vi "NT Table Connected AE.vi"(7 "Update":bool, 11 "NT Table Connected in":bool) -> (3 "NT Table Connected out":bool)   [LabVIEW 2025]
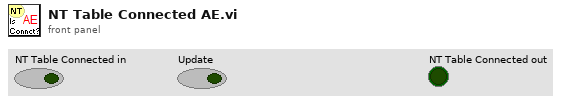
[diagram p1: front panel]
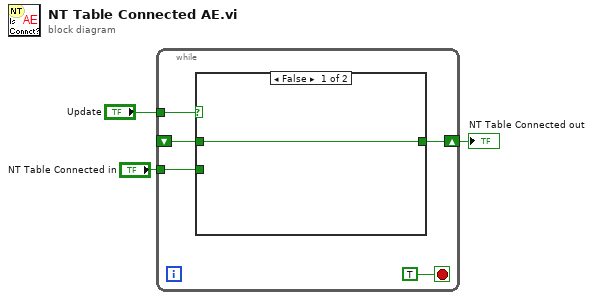
[diagram p0: block diagram]
diagram:
  n1 = while {
    shift-right: [w6] -> w1
    shift-left: _ -> [w4]
    tunnel: "Update" -> [w7]
    tunnel: "NT Table Connected in" -> [w5]
    stop <- TRUE stop-if-true
    n2 = case shown="False" w7 {
      tunnel: [w9 w10] -> w6
      tunnel: w5 -> [_ w10]
      tunnel: w4 -> [w9 _]
      frame False {
      }
      frame True {
      }
    }
  }
  "NT Table Connected out" <- w1
